vi "MoveRelSingleAxis.vi"(1 "Wait":bool=TRUE, 2 "Value":dbl format="%.2f", 3 "Axis":i32=1) -> (0 "Command executed":bool)   [LabVIEW 2019, in "DLLS4.lvclass"]
doc: "Move relative (single axis, 1..4)\nIf 'Wait' is set to 'true', the VI waits till the position is reached."
uses:
  Classes/Delay Line/DelayLineLS4/DLLS4.lvclass
  DLL/LStep4.dll
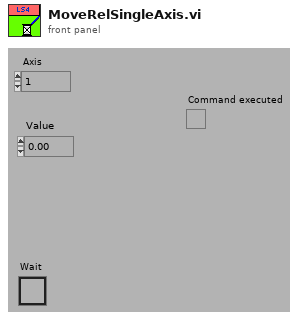
[diagram p1: front panel]
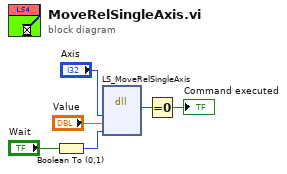
[diagram p0: block diagram]
diagram:
  n1 = Boolean To (0,1)(Boolean="Wait") -> (0, 1=w2:i16)
  n2 = dll-call lib="C:/Users/elysium/Documents/dev/TRANCON/DLL/LStep4.dll" fn="LS_MoveRelSingleAxis"("Axis"="Axis", "Value"="Value", "Wait"=w2) -> ("type de retour"=w4:i32)  [unwired: 6 in, 2 out]
  n3 = Equal To 0?(x=w4) -> (x = 0?=→"Command executed":bool)
